vi "Set RTDriver VIs File Paths.vi"(8 "error in (no error)":errorcluster, 11 "Item Ref in":T1 format="%.0x") -> (0 "error out":errorcluster, 3 "Item Ref out":T1 format="%.0x")   [LabVIEW 2021, in "gRPC Data Server System Explorer.lvlib"]
uses:
  gRPC Data Server System Explorer.lvlib
  <vilib>/NI VeriStand/Custom Device API/Custom Device Item Ref.ctl
  NationalInstruments.VeriStand.SystemDefinitionAPI
  NationalInstruments.VeriStand.SystemStorage
  <vilib>/Utility/LVLibp/NI_PackedLibraryUtility.lvlib
  <vilib>/NI VeriStand/Custom Device API/Custom Device API.lvlib
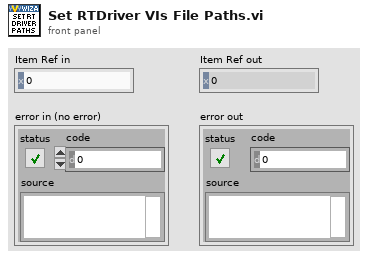
[diagram p1: front panel]
types:
  T1 = typedef "Custom Device API.lvlib/Custom Device Item Ref.ctl" = u64
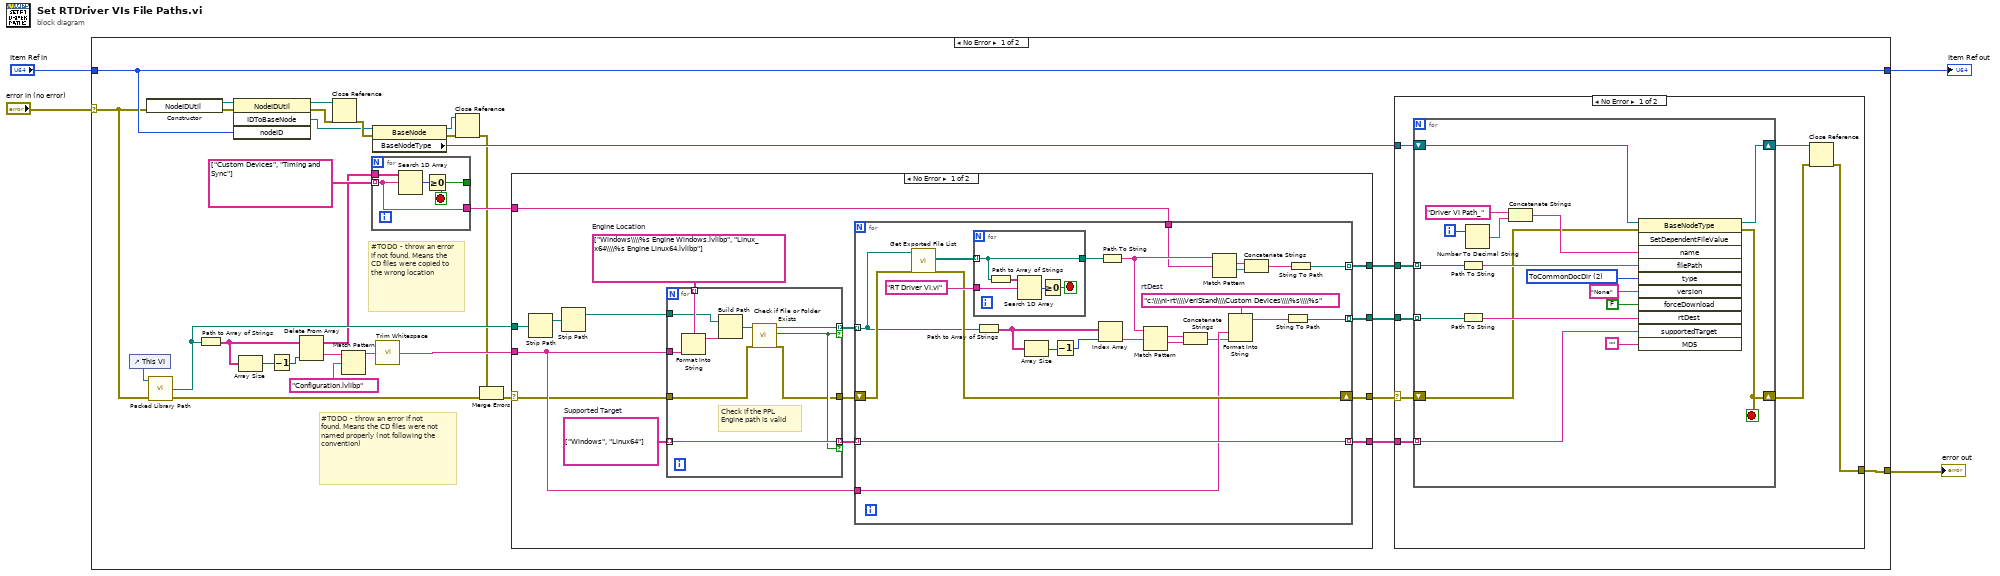
[diagram p0: block diagram]
diagram:
  n1 = case shown="No Error" "error in (no error)" {
    selector: "error in (no error)" -> [w13 w121]
    tunnel: [w35 w121] -> w4
    tunnel: [w26 w122] -> w3
    tunnel: "Item Ref in" -> [w26 w122]
    frame No Error {
      # "#TODO - throw an error if not found. Means the CD files were not named properly (not following the convention)"
      # "#TODO - throw an error if not found. Means the CD files were copied to the wrong location"
      n2 = control-ref of="This VI"() -> (w25:refnum<vi>)
      n3 = constructor class="NodeIDUtil"(error in=w13) -> (reference out=w27:refnum<k24>, error out=w28:errorcluster)  [unwired: 2 in, 1 out]
      n4 = call <vilib>:"Packed Library Path.vi"("error in (no error)"=w13, "vi reference"=w25) -> ("error out"=w6:errorcluster, "packed library path"=w24:path)  [unwired: 1 in, 1 out]
      n5 = Path to Array of Strings(0:w24) -> (2:w23:string[])  [unwired: 1 out]
      n6 = invoke class="NodeIDUtil" method="IDToBaseNode"(reference=w27, error in=w28, "nodeID"=w26) -> (reference out=w32:refnum<k24>, error out=w30:errorcluster, "IDToBaseNode"=w29:refnum<k24>)  [unwired: 1 in, 1 out]
      n7 = Array Size(array=w23) -> (size(s)=w22:i32)
      n8 = Decrement(x=w22) -> (x-1=w21:i32)
      n9 = Delete From Array(array=w23, index=w21) -> (deleted portion=w20:string, array with subset deleted=w16:string[])  [unwired: 1 in]
      n10 = Close Reference(reference=w32, error in (no error)=w30) -> (error out=w31:errorcluster)
      n11 = Match Pattern(string=w20, regular expression="Configuration.lvlibp") -> (before substring=w14:string)  [unwired: 1 in, 3 out]
      n12 = for {
        tunnel: string[] ["Custom Devices", "Timing and Sync"] ("array of strings") -> [w36] mode=indexing
        tunnel: [w38] -> _
        tunnel: w16 -> [w37]
        tunnel: [w36] -> w15
        stop <- w38 stop-if-true
        n13 = Search 1D Array(1D array=w37, element=w36) -> (index of element=w39:i32)  [unwired: 1 in]
        n14 = Greater Or Equal To 0?(x=w39) -> (x >= 0?=w38:bool)
      }
      n15 = property class="BaseNode"(reference=w29, error in=w31) -> (reference out=w33:refnum<k24>, error out=w34:errorcluster, "BaseNodeType"=w9:refnum<k24>)
      n16 = call <vilib>:"Trim Whitespace.vi"("string"=w14) -> ("trimmed string"=w18:string)  [unwired: 1 in]
      n17 = Close Reference(reference=w33, error in (no error)=w34) -> (error out=w5:errorcluster)
      n18 = Merge Errors(w5, w6) -> (w7:errorcluster)
      n19 = case shown="No Error" w7 {
        selector: w7 -> [w43 w94]
        tunnel: w24 -> [w53 _]
        tunnel: [w48 w94] -> w8
        tunnel: w18 -> [w44 _]
        tunnel: w15 -> [w52 _]
        tunnel: [w51 _] -> w12
        tunnel: [w50 _] -> w11
        tunnel: [w49 _] -> w10
        frame No Error {
          w47 = string[] ["Windows\\\\%s Engine Windows.lvlibp", "Linux_x64\\\\%s Engine Linux64.lvlibp"]  # Engine Location
          w45 = string[] ["Windows", "Linux64"]  # Supported Target
          n20 = Strip Path(path=w53) -> (stripped path=w54:path)  [unwired: 1 out]
          n21 = Strip Path(path=w54) -> (stripped path=w46:path)  [unwired: 1 out]
          n22 = for {
            tunnel: w47 -> [w64] mode=indexing
            tunnel: w46 -> [w62]
            tunnel: [w60] -> w40 mode=indexing if=w56
            tunnel: w43 -> [w57]
            tunnel: [w55] -> w42
            tunnel: w45 -> [w59] mode=indexing
            tunnel: [w59] -> w41 mode=indexing if=w56
            tunnel: w44 -> [w58]
            # "Check if the PPL Engine path is valid"
            n23 = Format Into String(format string=w64, w58) -> (resulting string=w63:string)  [unwired: 2 in, 1 out]
            n24 = Build Path(base path=w62, name or relative path=w63) -> (appended path=w61:path)
            n25 = call <vilib>:"Check if File or Folder Exists.vi"("error in (no error)"=w57, "path"=w61) -> ("error out"=w55:errorcluster, "file or folder exists?"=w56:bool, "dup path"=w60:path)  [unwired: 7 in]
          }
          n26 = for {
            shift-right: [w85] -> w48
            shift-left: w42 -> [w86]
            tunnel: w52 -> [w73]
            tunnel: [w72] -> w51 mode=indexing
            tunnel: [w71] -> w50 mode=indexing
            tunnel: [w70] -> w49 mode=indexing
            tunnel: w44 -> [w68]
            tunnel: w41 -> [w70] mode=indexing
            tunnel: w40 -> [w69] mode=indexing
            w65 = "c:\\\\ni-rt\\\\VeriStand\\\\Custom Devices\\\\%s\\\\%s"  # rtDest
            n27 = call <vilib>:"Get Exported File List.vi"("error in (no error)"=w86, "packed library path"=w69) -> ("error out"=w85:errorcluster, "paths"=w88:path[])  [unwired: 7 in, 1 out]
            n28 = for {
              tunnel: w88 -> [w90] mode=indexing
              tunnel: "RT Driver VI.vi" ("element") -> [w92]
              tunnel: [w90] -> w84
              stop <- w89 stop-if-true
              n29 = Path to Array of Strings(0:w90) -> (2:w93:string[])  [unwired: 1 out]
              n30 = Search 1D Array(1D array=w93, element=w92) -> (index of element=w91:i32)  [unwired: 1 in]
              n31 = Greater Or Equal To 0?(x=w91) -> (x >= 0?=w89:bool)
            }
            n32 = Path to Array of Strings(0:w69) -> (2:w76:string[])  [unwired: 1 out]
            n33 = Array Size(array=w76) -> (size(s)=w78:i32)
            n34 = Decrement(x=w78) -> (x-1=w77:i32)
            n35 = Index Array(array=w76, index=w77) -> (element=w75:string)
            n36 = Path To String(path=w84) -> (string=w81:string)
            n37 = Match Pattern(string=w81, regular expression=w75) -> (match substring=w80:string, after substring=w79:string)  [unwired: 1 in, 2 out]
            n38 = Concatenate Strings(w80, w79) -> (w67:string)
            n39 = Match Pattern(string=w81, regular expression=w73) -> (match substring=w83:string, after substring=w82:string)  [unwired: 1 in, 2 out]
            n40 = Format Into String(format string=w65, w68, w67) -> (resulting string=w66:string)  [unwired: 2 in, 1 out]
            n41 = Concatenate Strings(w83, w82) -> (w74:string)
            n42 = String To Path(string=w66) -> (path=w71:path)
            n43 = String To Path(string=w74) -> (path=w72:path)
          }
        }
        frame Error {
        }
      }
      n44 = case shown="No Error" w8 {
        selector: w8 -> [w96 w120]
        tunnel: [w101 w120] -> w35
        tunnel: w12 -> [w100 _]
        tunnel: w11 -> [w99 _]
        tunnel: w10 -> [w98 _]
        tunnel: w9 -> [w97 _]
        frame No Error {
          n45 = for {
            shift-right: [w106] -> w102
            shift-left: w97 -> [w114]
            tunnel: w100 -> [w111] mode=indexing
            tunnel: w99 -> [w110] mode=indexing
            tunnel: w98 -> [w109] mode=indexing
            shift-right: [w103] -> w95
            shift-left: w96 -> [w104]
            i -> [w118]
            stop <- w103 stop-if-true
            w113 = 2 items=["Absolute", "Relative", "ToCommonDocDir", "ToApplicationDataDir"] ("type")
            n46 = Path To String(path=w111) -> (string=w116:string)
            n47 = Path To String(path=w110) -> (string=w115:string)
            n48 = Number To Decimal String(number=w118) -> (decimal integer string=w119:string)  [unwired: 1 in]
            n49 = Concatenate Strings("Driver VI Path_" ("Property name"), w119) -> (w107:string)
            n50 = invoke class="BaseNodeType" method="SetDependentFileValue"(reference=w114, error in=w104, "name"=w107, "filePath"=w116, "type"=w113, "version"="None", "forceDownload"=FALSE, "rtDest"=w115, "supportedTarget"=w109, "MD5"="") -> (reference out=w106:refnum<k24>, error out=w103:errorcluster)  [unwired: 1 in, 9 out]
          }
          n51 = Close Reference(reference=w102, error in (no error)=w95) -> (error out=w101:errorcluster)
        }
        frame Error {
        }
      }
    }
    frame Error {
    }
  }
  "error out" <- w4
  "Item Ref out" <- w3
